vi "pump calibration.vi"(4 "pump ID":u8, 6 "pump cal command":T3=enum."Save default values", 8 "STAMP intercept":dbl, 9 "STAMP slope":dbl=2.52, 10 "flow rate":dbl[unit], 11 "Pump Calibration in":T1={"target 1"=0.0, "target 2"=0.0, "measured 1"=1e-06, "measured 2"=1e-06}) -> (0 "STAMP intercept out":dbl, 1 "STAMP slope out":dbl=2.52, 2 "modified flow rate":dbl[unit], 3 "Pump Calibration out":T1)   [LabVIEW 2012]
uses:
  calibration values.ctl
  calibration commands.ctl
  DAC project/Calibration and Function folders.ctl
  <vilib>/Utility/config.llb/Write Key (Double).vi
  <vilib>/Utility/config.llb/Read Key (Double).vi
  <vilib>/Utility/config.llb/NI_LVConfig.lvlib
panel:
  in  "pump calibrations default":T2(array[cluster])=[{"Pump Calibration"={"target 1"=0.0, "target 2"=1e-06, "measured 1"=0.0, "measured 2"=1e-06}, "STAMP slope"=1.0, "STAMP intercept"=0.0}, {"Pump Calibration"={"target 1"=0.0, "target 2"=1e-06, "measured 1"=0.0, "measured 2"=0.0}, "STAMP slope"=1.0, "STAMP intercept"=0.0}, {"Pump Calibration"={"target 1"=0.0, "target 2"=1e-06, "measured 1"=0.0, "measured 2"=0.0}, "STAMP slope"=1.0, "STAMP intercept"=0.0}, {"Pump Calibration"={"target 1"=0.0, "target 2"=1e-06, "measured 1"=0.0, "measured 2"=0.0}, "STAMP slope"=1.0, "STAMP intercept"=0.0}, {"Pump Calibration"={"target 1"=0.0, "target 2"=1e-06, "measured 1"=0.0, "measured 2"=0.0}, "STAMP slope"=1.0, "STAMP intercept"=0.0}, {"Pump Calibration"={"target 1"=0.0, "target 2"=1e-06, "measured 1"=0.0, "measured 2"=0.0}, "STAMP slope"=1.0, "STAMP intercept"=0.0}]
  out "pump calibrations":T2(array[cluster])
  in  "Pump Calibration default":T1={"target 1"=0.0, "target 2"=1e-06, "measured 1"=0.0, "measured 2"=1e-06}
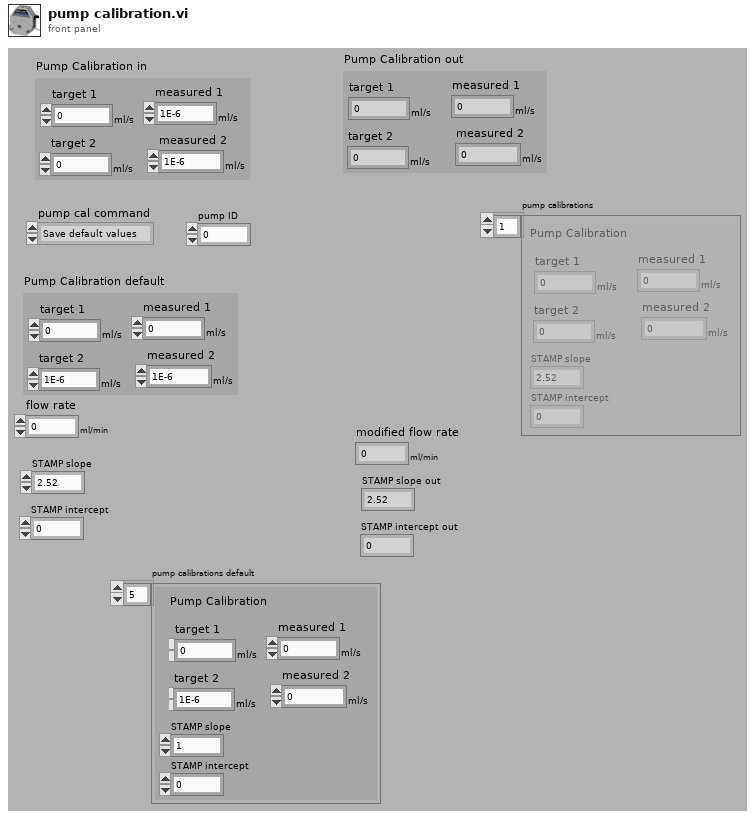
[diagram p1: front panel]
types:
  T1 = typedef "calibration values.ctl" = cluster{"target 1":dbl[unit], "target 2":dbl[unit], "measured 1":dbl[unit], "measured 2":dbl[unit]}
  T2 = cluster{"Pump Calibration":T1, "STAMP slope":dbl, "STAMP intercept":dbl}[]
  T3 = typedef "calibration commands.ctl" = enum16{"Get ini Path", "Save default values", "Save new calibration", "Read calibration", "Apply calibration", "Read STAMP mb", "Write STAMP mb"}
  T4 = typedef "Calibration and Function folders.ctl" = enum16{"Sensors", "Functions", "Config File", "UserAppFolder"}
  T5 = typedef "NI_LVConfig.lvlib/Config Data RefNum.ctl" = refnum<k1>
  T6 = cluster{"Pump Calibration":T1, "STAMP slope":dbl, "STAMP intercept":dbl}
  T7 = cluster{"[0]":dbl[unit], "[1]":dbl[unit], "[2]":dbl[unit], "[3]":dbl[unit]}
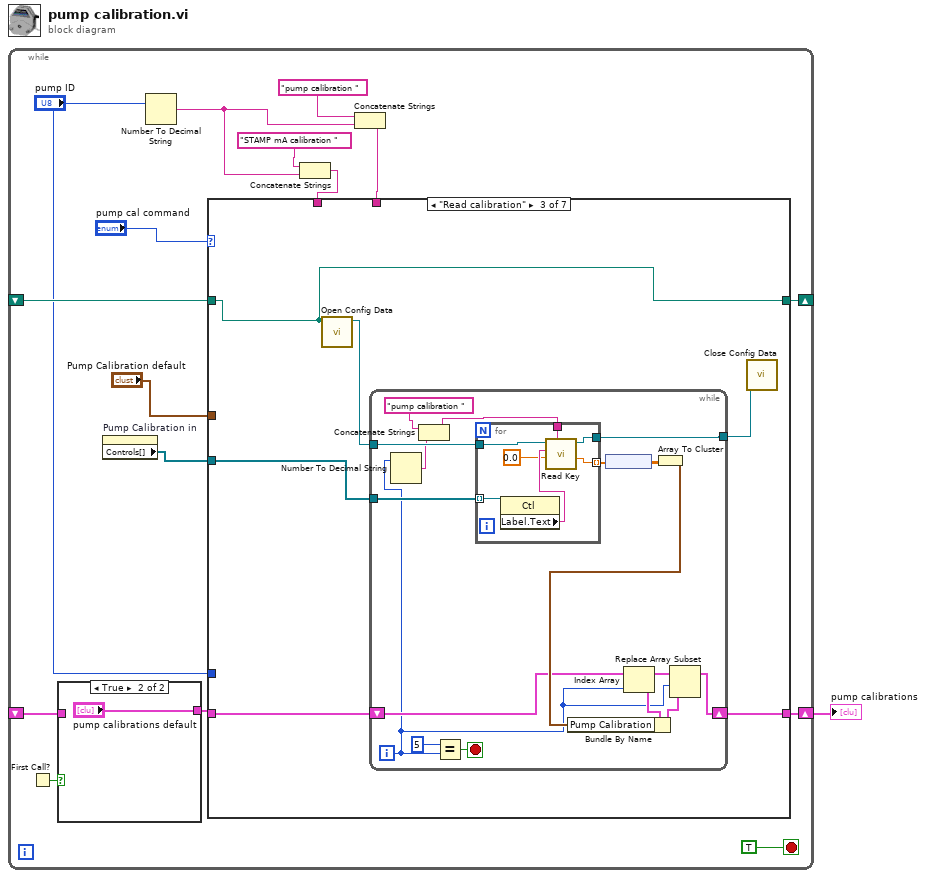
[diagram p0: block diagram]
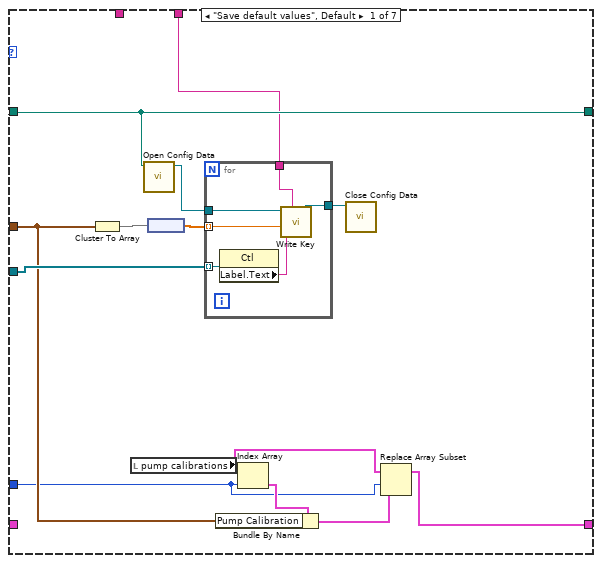
[diagram p3: hidden frame]
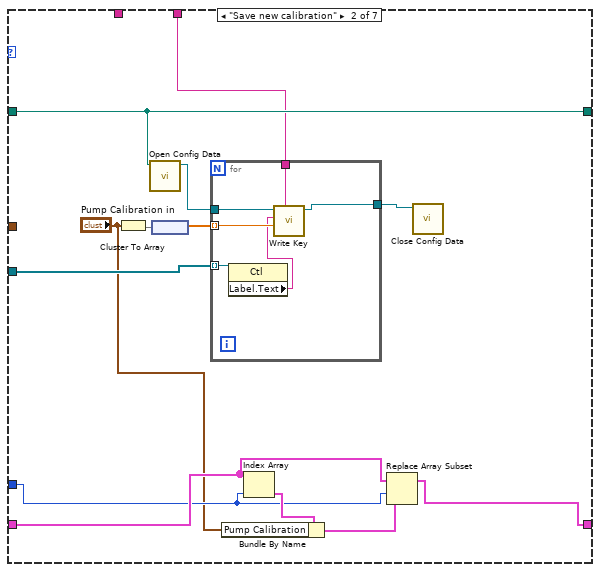
[diagram p4: hidden frame]
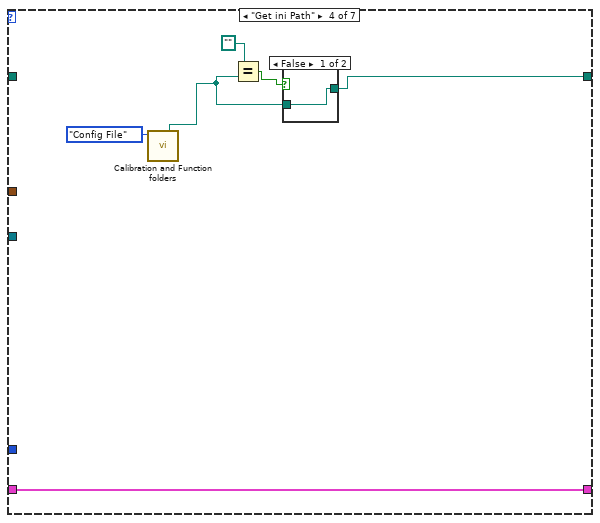
[diagram p5: hidden frame]
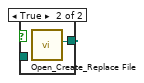
[diagram p6: hidden frame]
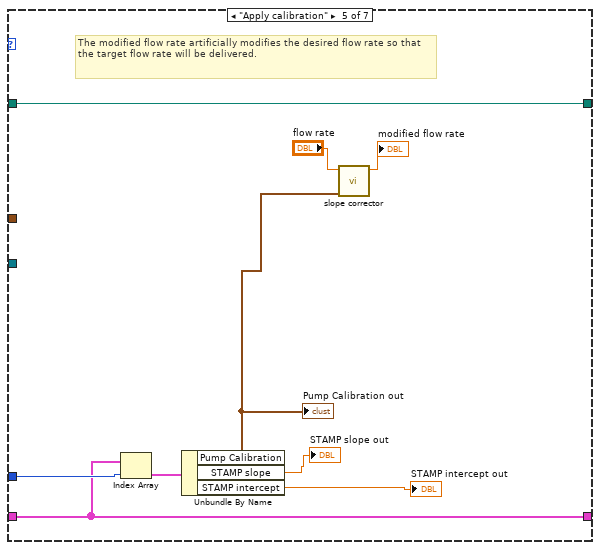
[diagram p7: hidden frame]
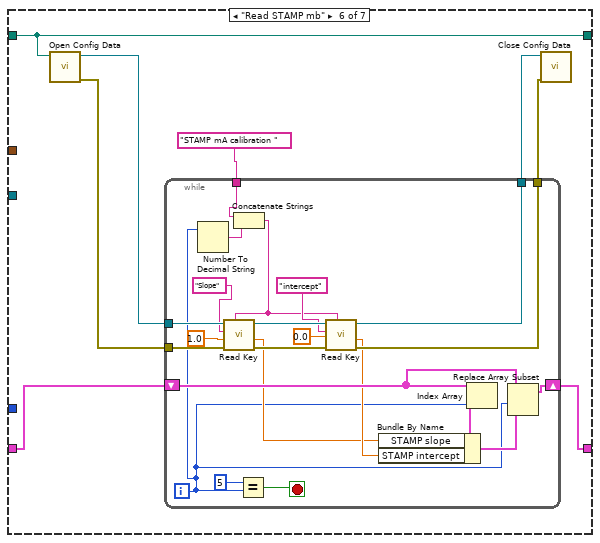
[diagram p8: hidden frame]
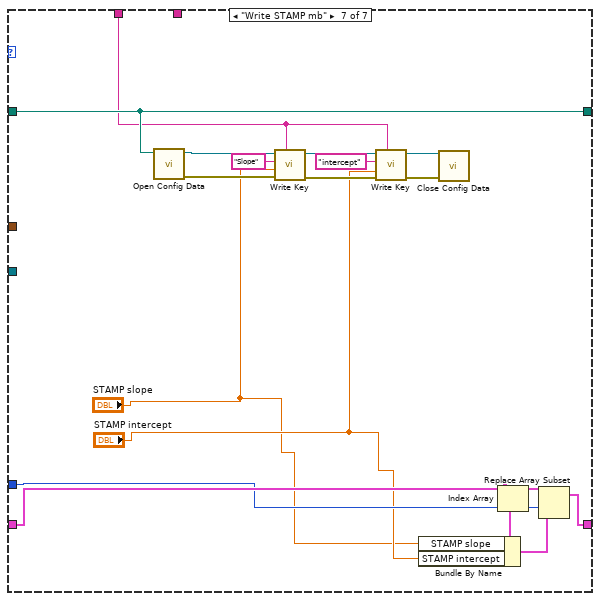
[diagram p9: hidden frame]
diagram:
  n1 = while {
    shift-right: [w14] -> _
    shift-left: _ -> [w16]
    shift-right: [w5] -> w1
    shift-left: _ -> [w3]
    stop <- TRUE stop-if-true
    n2 = First Call?() -> (First Call?: T/F=w4:bool)
    n3 = case shown="True" w4 {
      tunnel: w3 -> [w18 _]
      tunnel: [w18 "pump calibrations default"] -> w2
      frame False {
      }
      frame True {
      }
    }
    n4 = property on="Pump Calibration in" class="Clust (strict)"() -> ("Controls[]"=w15:refnum<vi>[])  [unwired: 2 in, 2 out]
    n5 = Number To Decimal String(number="pump ID") -> (decimal integer string=w8:string)  [unwired: 1 in]
    n6 = Concatenate Strings("STAMP mA calibration " ("section"), w8) -> (w7:string)
    n7 = Concatenate Strings("pump calibration " ("section"), w8) -> (w10:string)
    n8 = case shown="\"Read calibration\"" "pump cal command" {
      tunnel: w16 -> [w29 w49 w60 _ w103 w111 w150]
      tunnel: w15 -> [w28 w48 w61 _ _ _ _]
      tunnel: [w29 w49 w60 w90 w103 w111 w150] -> w14
      tunnel: w7 -> [_ _ _ _ _ _ w141]
      tunnel: w10 -> [w26 w45 _ _ _ _ _]
      tunnel: "Pump Calibration default" -> [w24 _ _ _ _ _ _]
      tunnel: "pump ID" -> [w22 w40 _ _ w100 _ w136]
      tunnel: [w20 w42 w58 w89 w99 w105 w138] -> w5
      tunnel: w2 -> [_ w41 w59 w89 w99 w106 w137]
      frame "Save default values", Default {
        n9 = Cluster To Array(cluster=w24) -> (array=w31:dbl[unit][])
        n10 = local read "pump calibrations"() -> (w23:T2)
        n11 = call <vilib>:"Open Config Data.vi"("configuration file path"=w29) -> ("refnum"=w32:T5)  [unwired: 8 in, 2 out]
        n12 = node(w31) -> (w27:dbl[])
        n13 = for {
          tunnel: w32 -> [w38]
          tunnel: w27 -> [w37] mode=indexing
          tunnel: w28 -> [w36] mode=indexing
          tunnel: w26 -> [w34]
          tunnel: [w33] -> w30
          n14 = property class="Ctl"(reference=w36) -> ("Label.Text"=w35:string)  [unwired: 1 in, 2 out]
          n15 = call-poly <vilib>:"Write Key.vi"("section"=w34, "value"=w37, "key"=w35, "refnum"=w38) -> ("refnum out"=w33:T5)  [unwired: 5 in, 2 out]
        }
        n16 = Index Array(array=w23, index=w22) -> (element=w25:T6)
        n17 = Bundle By Name(cluster=w25, "Pump Calibration"=w24) -> (w21:T6)
        n18 = call <vilib>:"Close Config Data.vi"("refnum"=w30) -> ()  [unwired: 9 in, 2 out]
        n19 = Replace Array Subset(array=w23, new element=w21, index=w22) -> (w20:T2)
      }
      frame "Save new calibration" {
        n20 = Cluster To Array(cluster="Pump Calibration in") -> (array=w46:dbl[unit][])
        n21 = call <vilib>:"Open Config Data.vi"("configuration file path"=w49) -> ("refnum"=w51:T5)  [unwired: 8 in, 2 out]
        n22 = node(w46) -> (w47:dbl[])
        n23 = for {
          tunnel: w51 -> [w57]
          tunnel: w47 -> [w56] mode=indexing
          tunnel: w48 -> [w55] mode=indexing
          tunnel: w45 -> [w53]
          tunnel: [w52] -> w50
          n24 = property class="Ctl"(reference=w55) -> ("Label.Text"=w54:string)  [unwired: 1 in, 2 out]
          n25 = call-poly <vilib>:"Write Key.vi"("section"=w53, "value"=w56, "key"=w54, "refnum"=w57) -> ("refnum out"=w52:T5)  [unwired: 5 in, 2 out]
        }
        n26 = Index Array(array=w41, index=w40) -> (element=w44:T6)
        n27 = Bundle By Name(cluster=w44, "Pump Calibration"="Pump Calibration in") -> (w43:T6)
        n28 = Replace Array Subset(array=w41, new element=w43, index=w40) -> (w42:T2)
        n29 = call <vilib>:"Close Config Data.vi"("refnum"=w50) -> ()  [unwired: 9 in, 2 out]
      }
      frame "Read calibration" {
        n30 = call <vilib>:"Open Config Data.vi"("configuration file path"=w60) -> ("refnum"=w63:T5)  [unwired: 8 in, 2 out]
        n31 = while {
          tunnel: w63 -> [w79]
          tunnel: [w78] -> w62
          tunnel: w61 -> [w76]
          shift-right: [w70] -> w58
          shift-left: w59 -> [w71]
          i -> [w66]
          stop <- w64 stop-if-true
          n32 = Number To Decimal String(number=w66) -> (decimal integer string=w68:string)  [unwired: 1 in]
          n33 = Concatenate Strings("pump calibration " ("section"), w68) -> (w67:string)
          n34 = Equal?(x=5, y=w66) -> (x = y?=w64:bool)
          n35 = for {
            tunnel: w79 -> [w86]
            tunnel: w76 -> [w85] mode=indexing
            tunnel: w67 -> [w83]
            tunnel: [w82] -> w78
            tunnel: [w80] -> w77 mode=indexing
            n36 = property class="Ctl"(reference=w85) -> ("Label.Text"=w84:string)  [unwired: 1 in, 2 out]
            n37 = call-poly <vilib>:"Read Key.vi"("section"=w83, "default value"=0.0 ("target 1"), "key"=w84, "refnum"=w86) -> ("value"=w80:dbl, "refnum out"=w82:T5)  [unwired: 4 in, 2 out]
          }
          n38 = node(w77) -> (w75:dbl[unit][])
          n39 = Index Array(array=w71, index=w66) -> (element=w74:T6)
          n40 = Array To Cluster(array=w75) -> (cluster=w72:T7)
          n41 = Bundle By Name(cluster=w74, "Pump Calibration"=w72) -> (w73:T6)
          n42 = Replace Array Subset(array=w71, new element=w73, index=w66) -> (w70:T2)
        }
        n43 = call <vilib>:"Close Config Data.vi"("refnum"=w62) -> ()  [unwired: 9 in, 2 out]
      }
      frame "Get ini Path" {
        n44 = call "Calibration and Function folders.vi"("Folder"=Calibration_and_Function_folders."Config File") -> ("Selected Folder"=w87:path)  [unwired: 10 in]
        n45 = Equal?(x=path "", y=w87) -> (x = y?=w92:bool)
        n46 = case shown="False" w92 {
          tunnel: [w93 w94] -> w90
          tunnel: w87 -> [w93 _]
          frame False {
          }
          frame True {
            n47 = call <vilib>:"Open_Create_Replace File.vi"() -> ("new file path"=w94:path)  [unwired: 8 in, 3 out]
          }
        }
      }
      frame "Apply calibration" {
        # "The modified flow rate artificially modifies the desired flow rate so that the target flow rate will be delivered."
        n48 = Index Array(array=w99, index=w100) -> (element=w98:T6)
        n49 = Unbundle By Name(w98) -> ("Pump Calibration"=w95:T1, "STAMP slope"=→"STAMP slope out":dbl, "STAMP intercept"=→"STAMP intercept out":dbl)
        "Pump Calibration out" <- w95
        n50 = call "slope corrector.vi"("Pump Calibration"=w95, "flow rate"="flow rate") -> ("modified flow rate"=→"modified flow rate":dbl[unit])  [unwired: 9 in]
      }
      frame "Read STAMP mb" {
        n51 = call <vilib>:"Open Config Data.vi"("configuration file path"=w111) -> ("error out"=w108:errorcluster, "refnum"=w110:T5)  [unwired: 8 in, 1 out]
        n52 = while {
          tunnel: w110 -> [w133]
          tunnel: [w131] -> w109
          tunnel: w108 -> [w130]
          tunnel: [w128] -> w107
          shift-right: [w119] -> w105
          shift-left: w106 -> [w122]
          tunnel: "STAMP mA calibration " ("section") -> [w116]
          i -> [w114]
          stop <- w112 stop-if-true
          n53 = Number To Decimal String(number=w114) -> (decimal integer string=w115:string)  [unwired: 1 in]
          n54 = Concatenate Strings(w116, w115) -> (w117:string)
          n55 = call-poly <vilib>:"Read Key.vi"("section"=w117, "error in (no error)"=w130, "default value"=1.0 ("STAMP slope"), "key"="Slope", "refnum"=w133) -> ("error out"=w129:errorcluster, "value"=w120:dbl, "refnum out"=w132:T5)  [unwired: 3 in, 1 out]
          n56 = Equal?(x=5, y=w114) -> (x = y?=w112:bool)
          n57 = call-poly <vilib>:"Read Key.vi"("section"=w117, "error in (no error)"=w129, "default value"=0.0 ("STAMP intercept"), "key"="intercept", "refnum"=w132) -> ("error out"=w128:errorcluster, "value"=w121:dbl, "refnum out"=w131:T5)  [unwired: 3 in, 1 out]
          n58 = Index Array(array=w122, index=w114) -> (element=w124:T6)
          n59 = Bundle By Name(cluster=w124, "STAMP slope"=w120, "STAMP intercept"=w121) -> (w123:T6)
          n60 = Replace Array Subset(array=w122, new element=w123, index=w114) -> (w119:T2)
        }
        n61 = call <vilib>:"Close Config Data.vi"("error in (no error)"=w107, "refnum"=w109) -> ()  [unwired: 8 in, 2 out]
      }
      frame "Write STAMP mb" {
        n62 = call <vilib>:"Open Config Data.vi"("configuration file path"=w150) -> ("error out"=w144:errorcluster, "refnum"=w149:T5)  [unwired: 8 in, 1 out]
        n63 = call-poly <vilib>:"Write Key.vi"("section"=w141, "error in (no error)"=w144, "value"="STAMP slope", "key"="Slope", "refnum"=w149) -> ("error out"=w143:errorcluster, "refnum out"=w148:T5)  [unwired: 4 in, 1 out]
        n64 = call-poly <vilib>:"Write Key.vi"("section"=w141, "error in (no error)"=w143, "value"="STAMP intercept", "key"="intercept", "refnum"=w148) -> ("error out"=w142:errorcluster, "refnum out"=w147:T5)  [unwired: 4 in, 1 out]
        n65 = call <vilib>:"Close Config Data.vi"("error in (no error)"=w142, "refnum"=w147) -> ()  [unwired: 8 in, 2 out]
        n66 = Index Array(array=w137, index=w136) -> (element=w140:T6)
        n67 = Bundle By Name(cluster=w140, "STAMP slope"="STAMP slope", "STAMP intercept"="STAMP intercept") -> (w139:T6)
        n68 = Replace Array Subset(array=w137, new element=w139, index=w136) -> (w138:T2)
      }
    }
  }
  "pump calibrations" <- w1
